vi "Pre-Build Custom Action.vi"(10 "Variant":variant) -> (0 "error out":errorcluster)   [LabVIEW 2017]
panel:
  out "States Out":string
  out "Current State":string
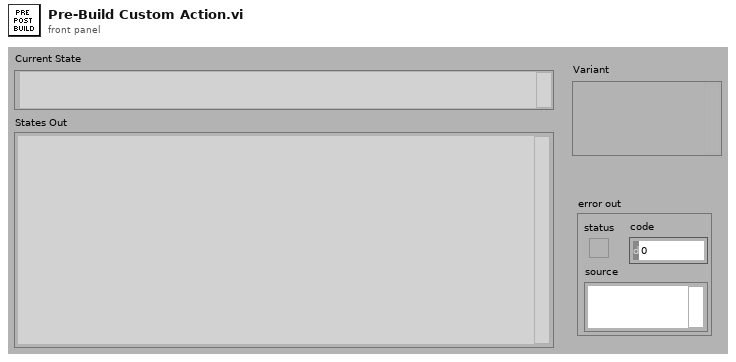
[diagram p1: front panel]
types:
  T1 = enum32{"Invalid", "Standard", "Closed", "Hidden", "Minimized", "Maximized"}
  T2 = enum32{"invalid app kind", "Development System", "Run Time System", "Student Edition", "Embedded LabVIEW", "Evaluation", "Custom"}
  T3 = cluster{"Core":cluster{"Current VI Reference":refnum<vi>, "Close Panel on Exit?":bool}, "Your Boolean data":bool, "Your string data":string}
  T4 = cluster{"Current VI Reference":refnum<vi>, "Close Panel on Exit?":bool}
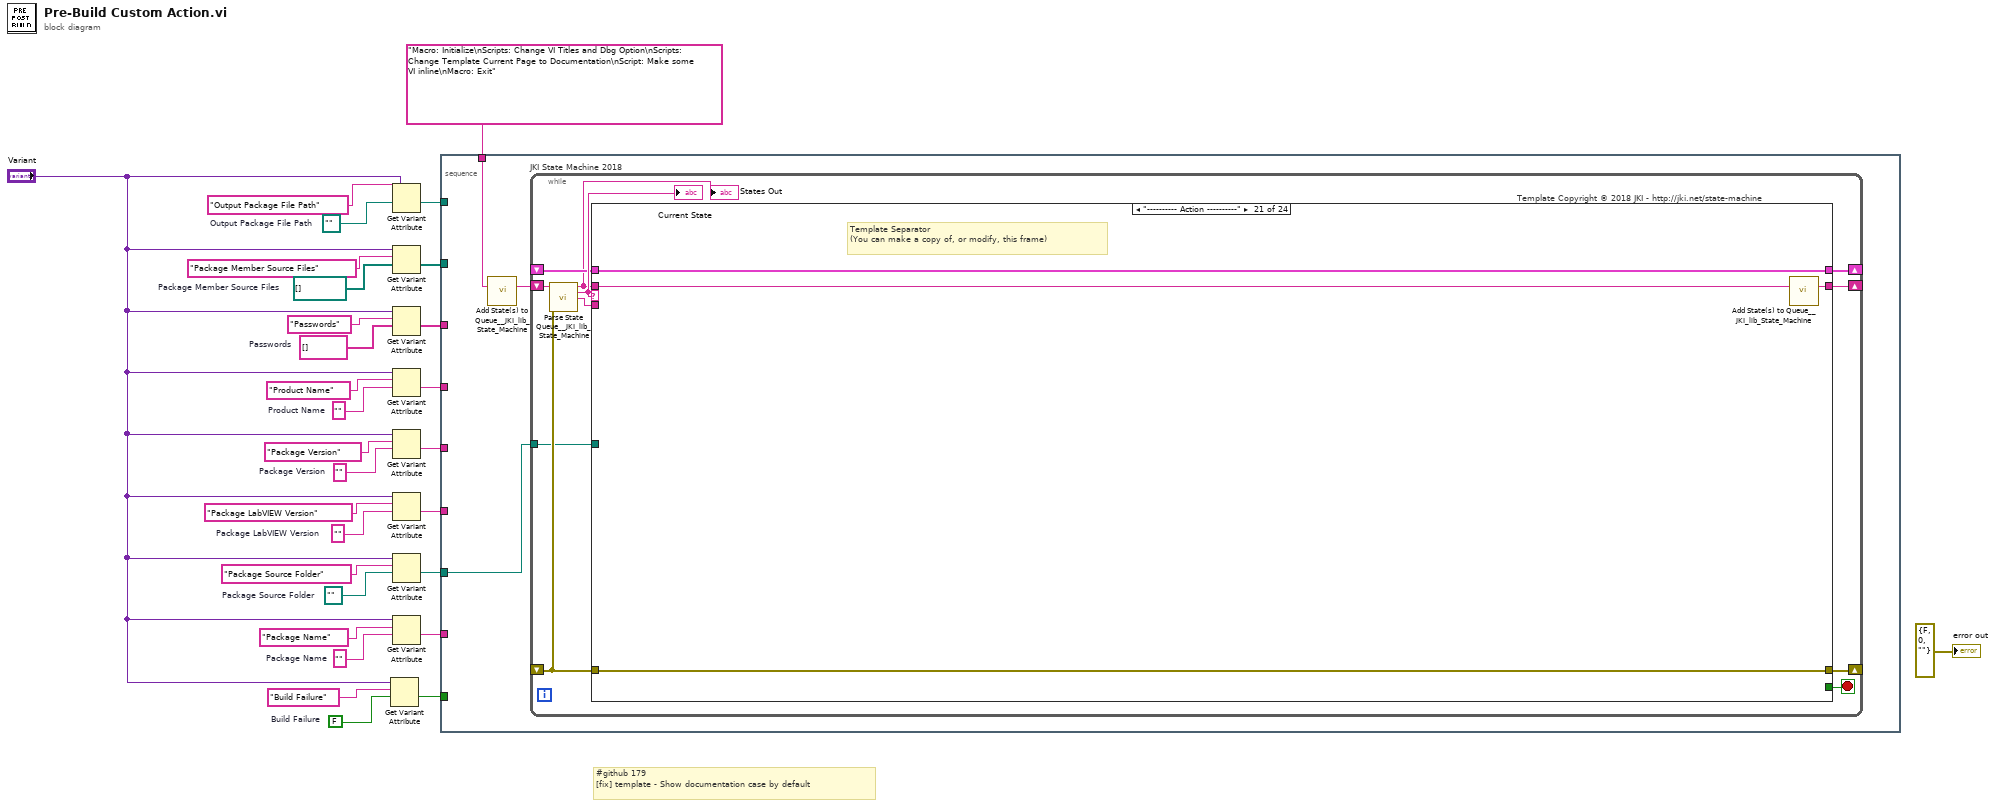
[diagram p0: block diagram]
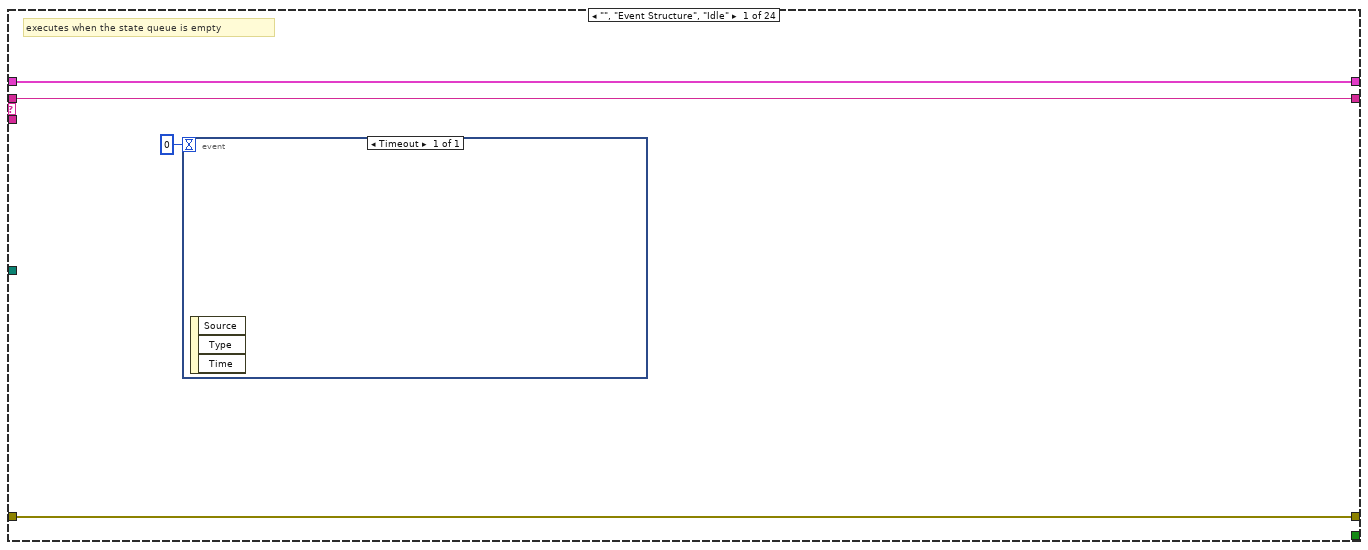
[diagram p2: hidden frame]
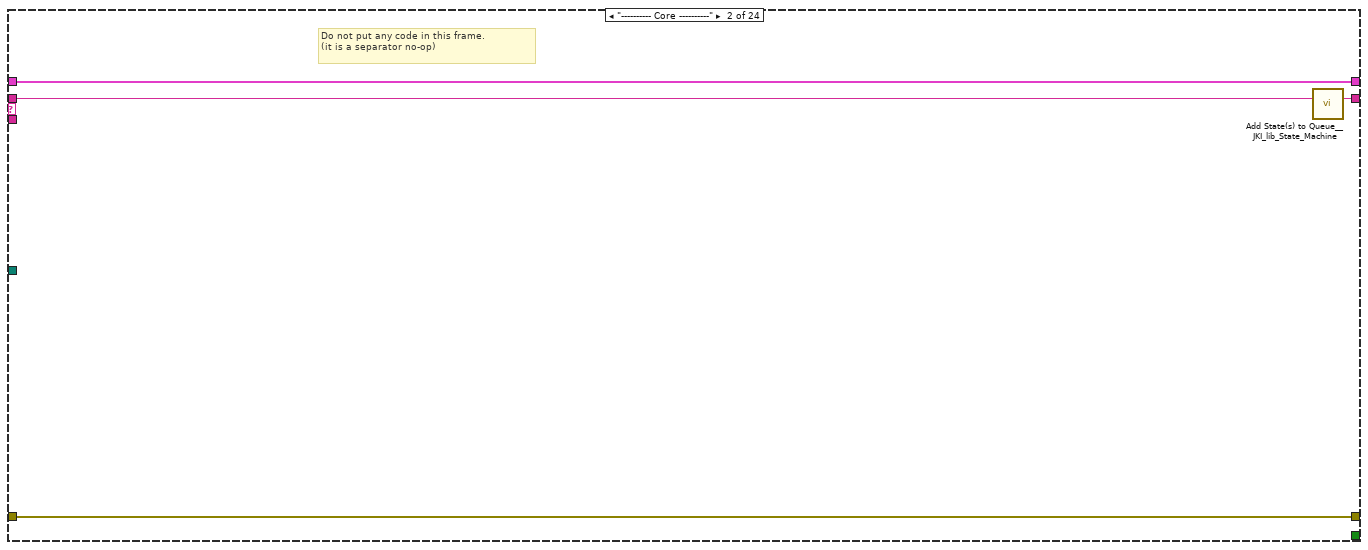
[diagram p3: hidden frame]
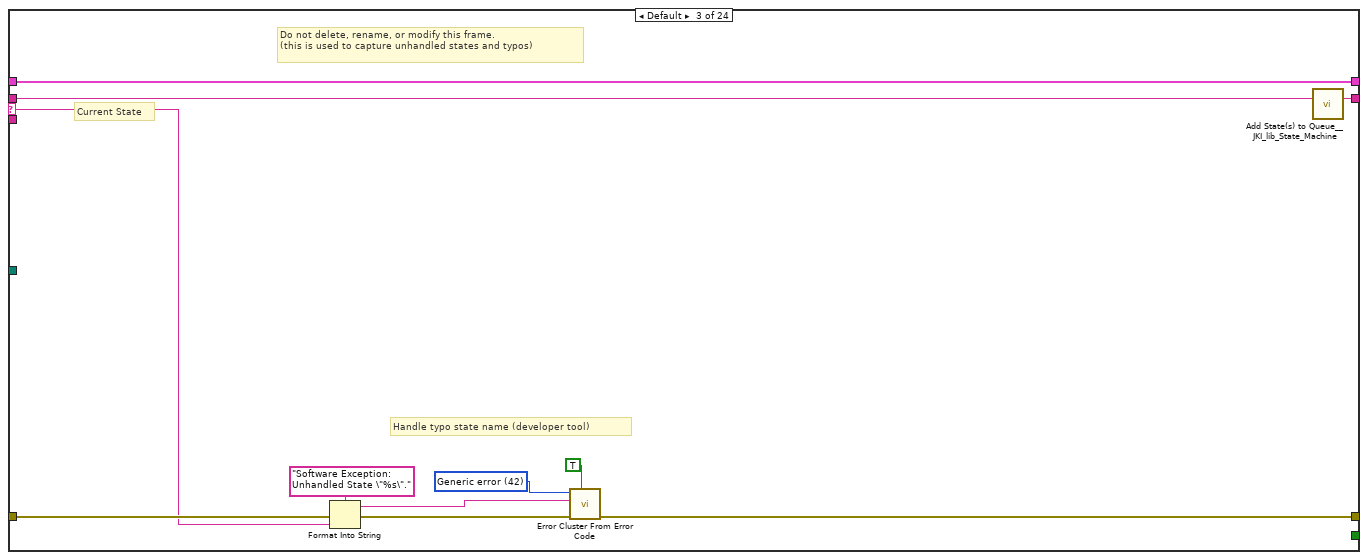
[diagram p4: hidden frame]
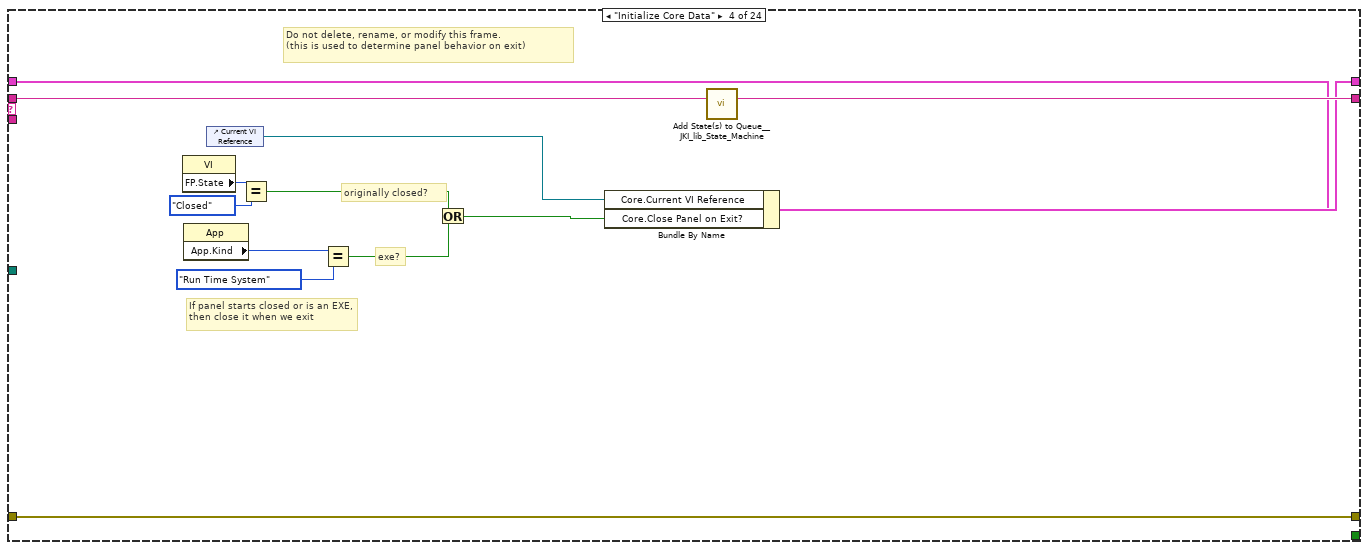
[diagram p5: hidden frame]
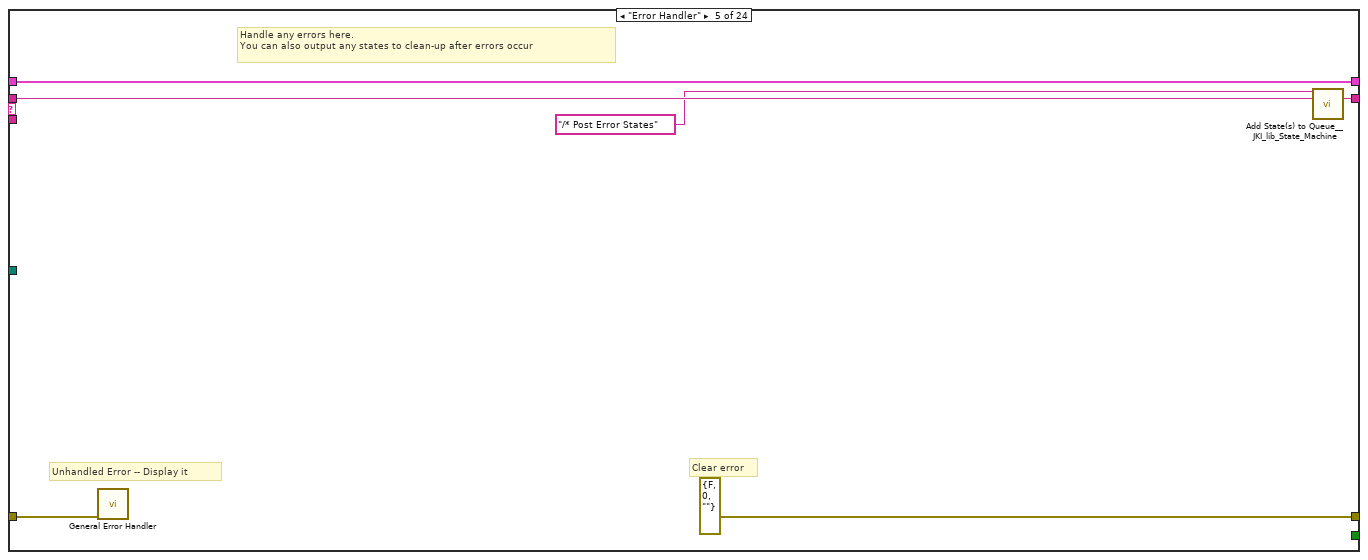
[diagram p6: hidden frame]
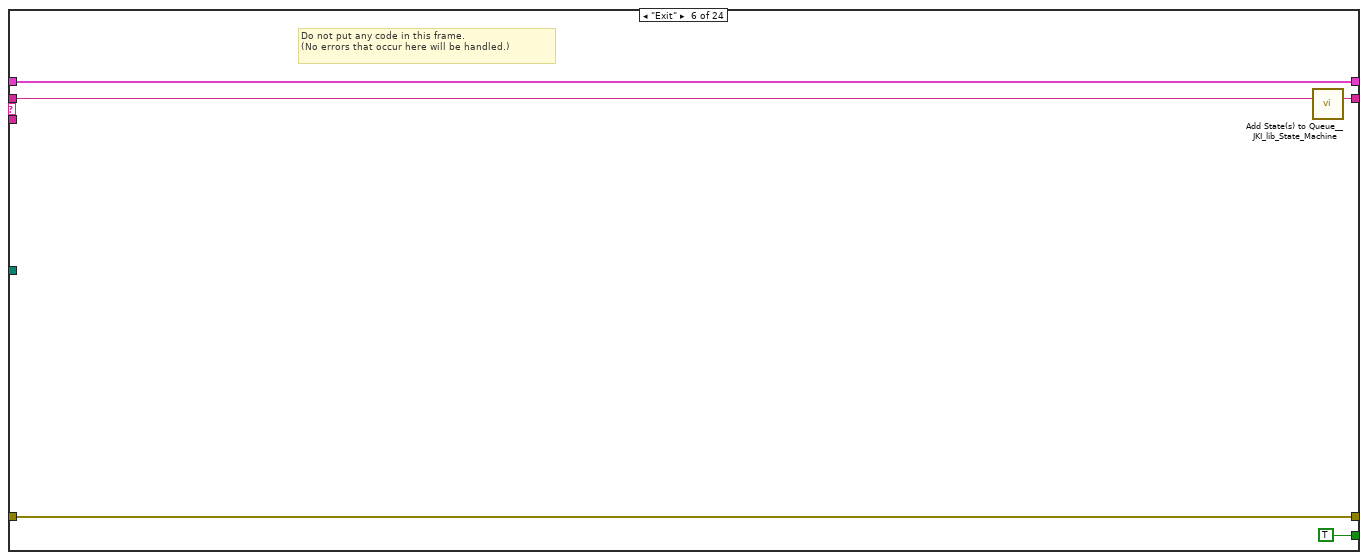
[diagram p7: hidden frame]
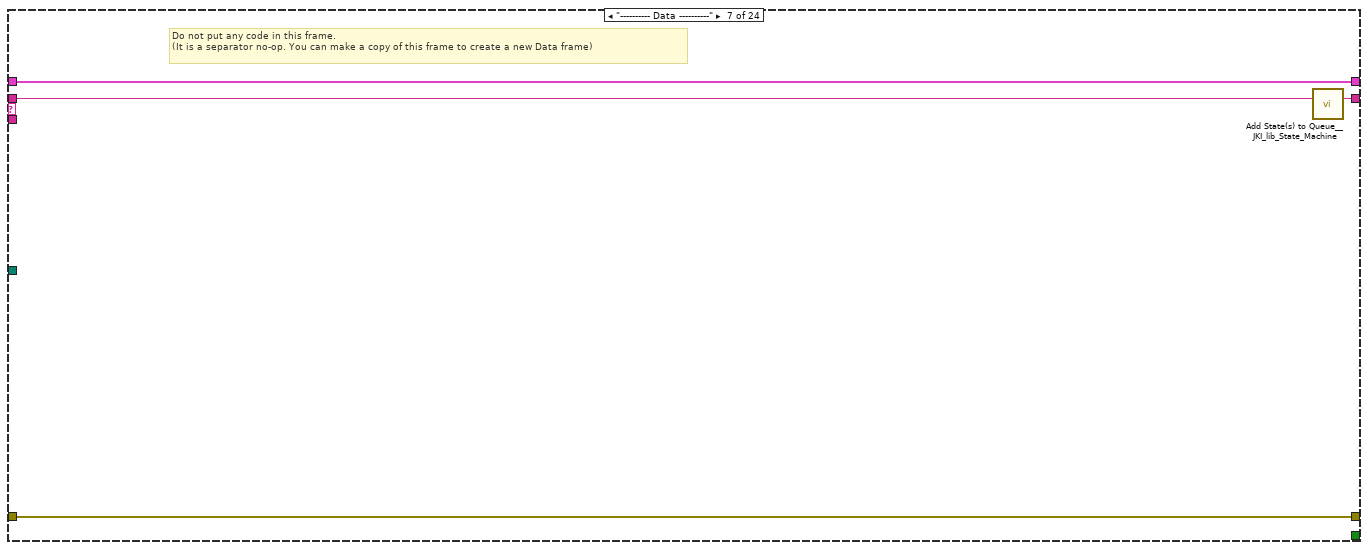
[diagram p8: hidden frame]
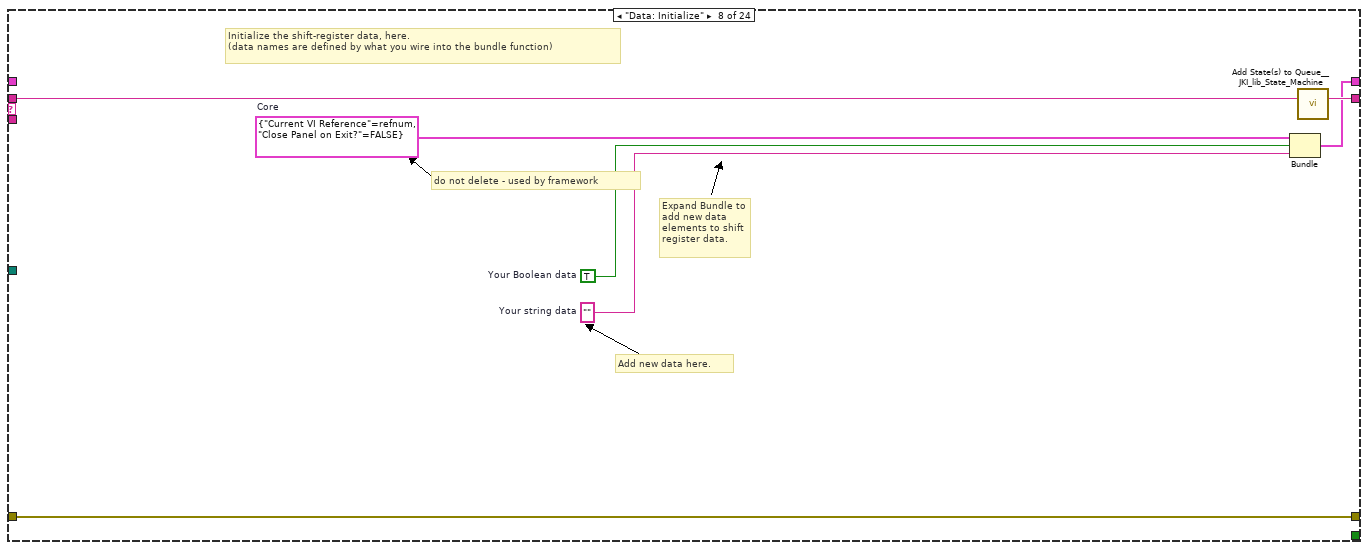
[diagram p9: hidden frame]
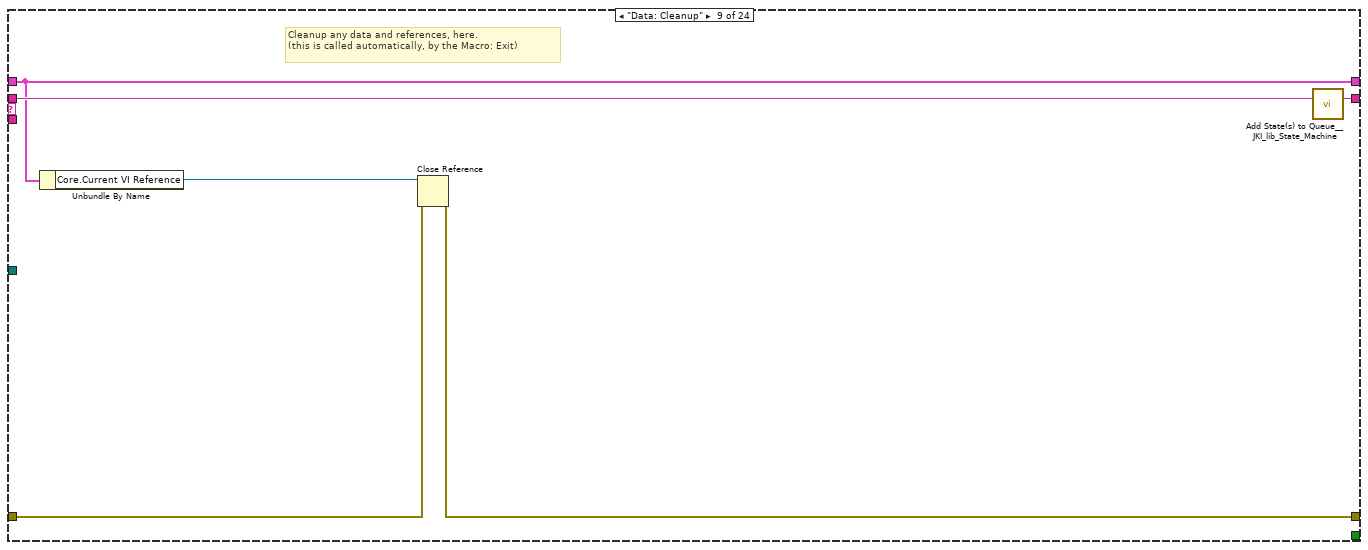
[diagram p10: hidden frame]
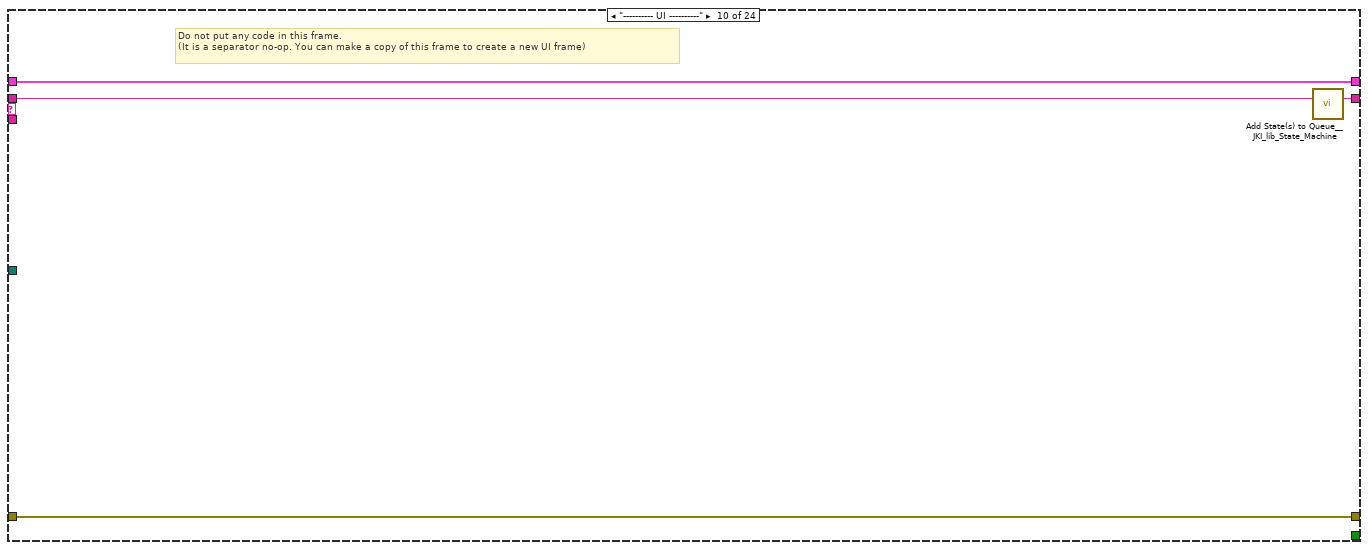
[diagram p11: hidden frame]
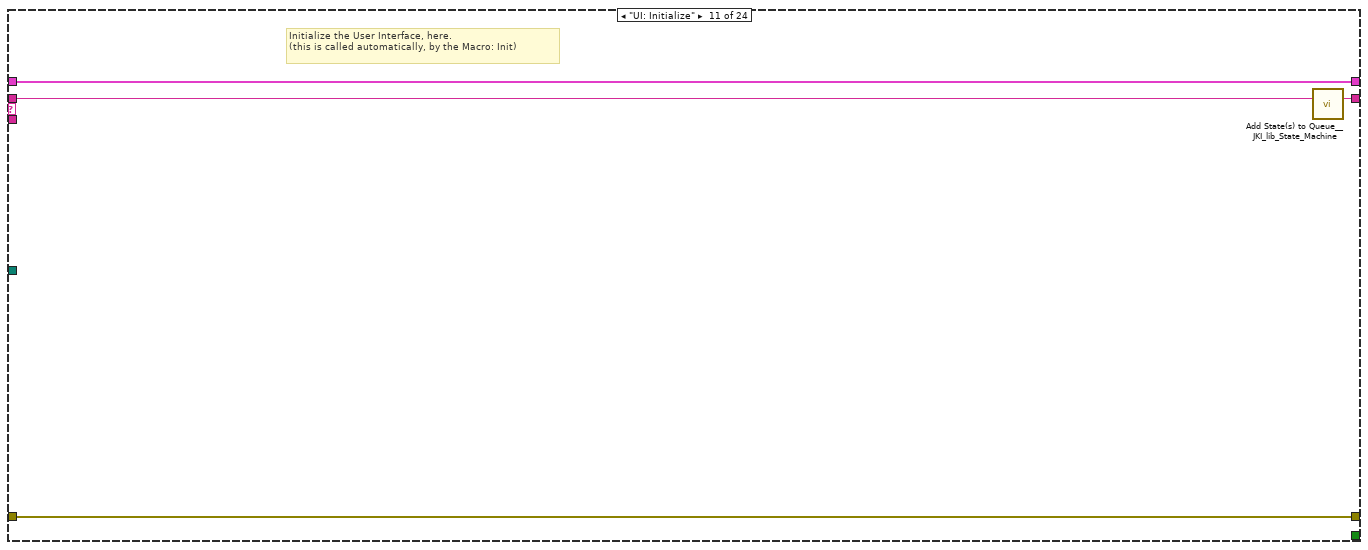
[diagram p12: hidden frame]
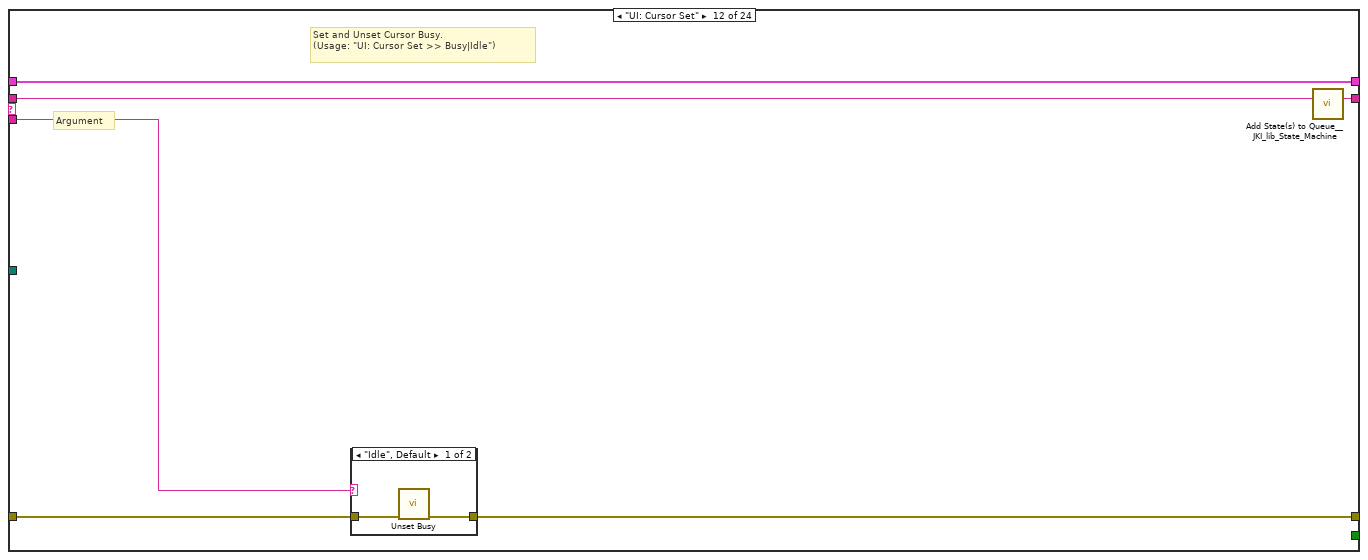
[diagram p13: hidden frame]
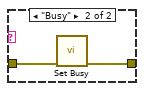
[diagram p14: hidden frame]
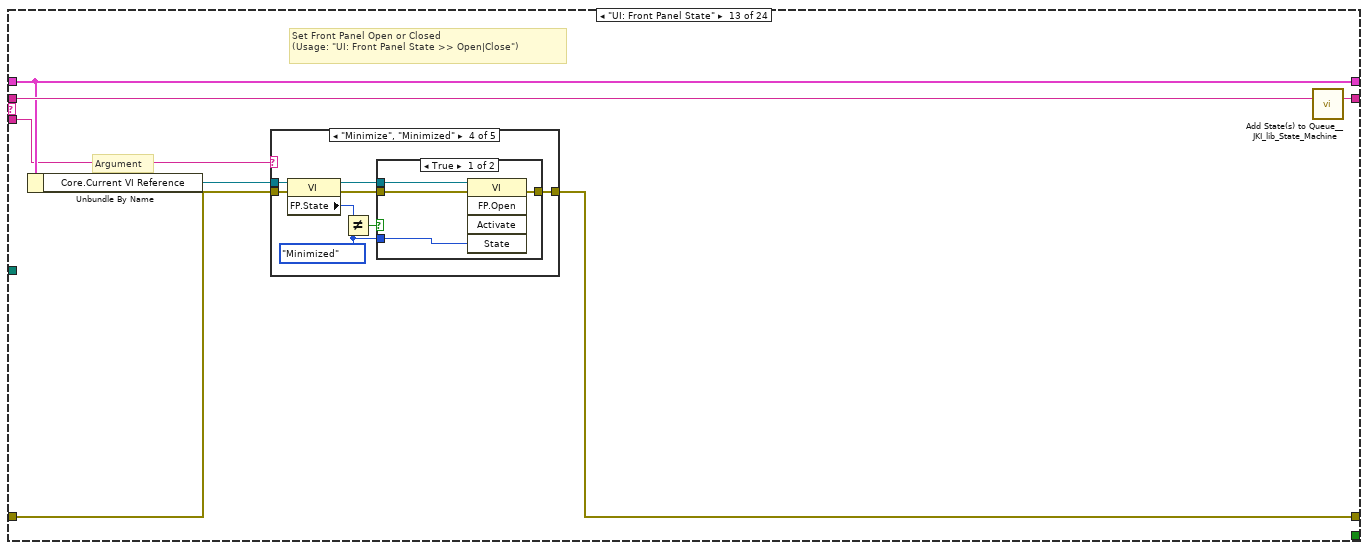
[diagram p15: hidden frame]
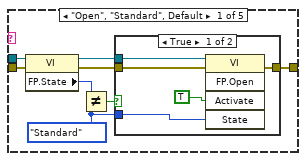
[diagram p16: hidden frame]
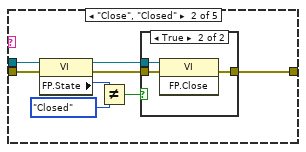
[diagram p18: hidden frame]
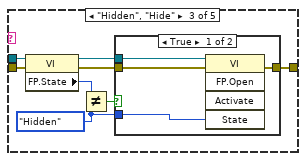
[diagram p20: hidden frame]
diagram:
  w4 = FALSE  # Build Failure
  w14 = path ""  # Package Source Folder
  w15 = ""  # Package Name
  w18 = ""  # Package LabVIEW Version
  w20 = ""  # Package Version
  w22 = ""  # Product Name
  w25 = string[] []  # Passwords
  w27 = path[] []  # Package Member Source Files
  w29 = path ""  # Output Package File Path
  # "#github 179\n[fix] template - Show documentation case by default"
  n1 = Get Variant Attribute(Variant="Variant", name="Build Failure", default value (empty Variant)=w4) -> (value=w2:bool)  [unwired: 1 in, 3 out]
  n2 = Get Variant Attribute(Variant="Variant", name="Output Package File Path", default value (empty Variant)=w29) -> (value=w13:path)  [unwired: 1 in, 3 out]
  n3 = Get Variant Attribute(Variant="Variant", name="Package Member Source Files", default value (empty Variant)=w27) -> (value=w12:path[])  [unwired: 1 in, 3 out]
  n4 = Get Variant Attribute(Variant="Variant", name="Passwords", default value (empty Variant)=w25) -> (value=w11:string[])  [unwired: 1 in, 3 out]
  n5 = Get Variant Attribute(Variant="Variant", name="Product Name", default value (empty Variant)=w22) -> (value=w10:string)  [unwired: 1 in, 3 out]
  n6 = Get Variant Attribute(Variant="Variant", name="Package Version", default value (empty Variant)=w20) -> (value=w9:string)  [unwired: 1 in, 3 out]
  n7 = Get Variant Attribute(Variant="Variant", name="Package LabVIEW Version", default value (empty Variant)=w18) -> (value=w8:string)  [unwired: 1 in, 3 out]
  n8 = Get Variant Attribute(Variant="Variant", name="Package Source Folder", default value (empty Variant)=w14) -> (value=w7:path)  [unwired: 1 in, 3 out]
  n9 = Get Variant Attribute(Variant="Variant", name="Package Name", default value (empty Variant)=w15) -> (value=w6:string)  [unwired: 1 in, 3 out]
  n10 = stacked-sequence {
    tunnel: w13 -> [_]
    tunnel: w12 -> [_]
    tunnel: w11 -> [_]
    tunnel: w10 -> [_]
    tunnel: w9 -> [_]
    tunnel: w8 -> [_]
    tunnel: w7 -> [w32]
    tunnel: w6 -> [_]
    tunnel: w2 -> [_]
    tunnel: "Macro: Initialize\nScripts: Change VI Titles and Dbg Option\nScripts: Change Template Current Page to Documentation\nScript: Make some VI inline\nMacro: Exit" -> [w31]
    frame #0 {
      n11 = call <vilib>:"Add State(s) to Queue__JKI_lib_State_Machine.vi"("State(s) in (\"\")"=w31) -> ("States Out"=w33:string)  [unwired: 14 in]
      n12 = while "JKI State Machine 2018" {
        shift-right: [w38] -> _
        shift-left: _ -> [w37]
        shift-right: [w41] -> _
        shift-left: _ -> [w36]
        shift-right: [w40] -> _
        shift-left: w33 -> [w42]
        tunnel: w32 -> [w35]
        stop <- w39 stop-if-true
        # "Template Copyright © 2018 JKI - http://jki.net/state-machine"
        n13 = call <vilib>:"Parse State Queue__JKI_lib_State_Machine.vi"("State Queue"=w42, "Error In (no error)"=w36) -> ("Remaining States"=w34:string, "Current State"=w44:string, "Arguments"=w43:string)  [unwired: 11 in]
        "Current State" <- w44
        "States Out" <- w34
        n14 = case shown="\"---------- Action ----------\"" w44 {
          selector: w44 -> [_ _ w53 _ _ _ _ _ _ _ _ _ _ _ _ _ _ _ _ _ _ _ _ _]
          tunnel: w34 -> [w47 w52 w57 w76 w82 w87 w91 w98 w104 w108 w112 w118 w129 w198 w203 w213 w217 w225 w265 w288 w312 w350 w375 w411]
          tunnel: w43 -> [_ _ _ _ _ _ _ _ _ _ _ w113 w123 _ _ _ _ _ _ _ _ w313 w357 w405]
          tunnel: w37 -> [w48 w49 w55 w69 w79 w85 w88 _ w99 w105 w110 w116 w125 w195 w200 w210 w214 w230 w268 w292 w309 w347 w372 w408]
          tunnel: [w46 w50 w59 w73 errorcluster {"status"=FALSE, "code"=0, "source"=""} ("error out") w84 w89 w95 w100 w106 w109 w114 w126 w196 w201 w211 w215 w231 w269 w293 w310 w348 w373 w409] -> w41
          tunnel: w36 -> [w46 w50 w58 w73 w78 w84 w89 w95 w101 w106 w109 w115 w127 w196 w201 w211 w215 w231 w269 w293 w310 w348 w373 w409]
          tunnel: [w47 w51 w56 w75 w81 w86 w90 w97 w103 w107 w111 w117 w128 w197 w202 w212 w216 w224 w264 w287 w311 w349 w374 w410] -> w40
          tunnel: [_ _ _ _ _ TRUE _ _ _ _ _ _ _ _ _ _ _ _ _ _ _ _ _ _] -> w39
          tunnel: [w48 w49 w55 w74 w79 w85 w88 w96 w99 w105 w110 w116 w125 w195 w200 w210 w214 w230 w268 w292 w309 w347 w372 w408] -> w38
          tunnel: w35 -> [_ _ _ _ _ _ _ _ _ _ _ _ _ _ _ _ _ w227 w267 w290 _ _ _ _]
          frame "", "Event Structure", "Idle" {
            # "executes when the state queue is empty"
            n15 = event shown="[0] Timeout" {
              selector: _ -> [_]
              dyn-events: _ -> [_]
              timeout: 0 -> [_]
              event Timeout {
                n16 = event-data() -> ()  [unwired: 1 in, 3 out]
              }
            }
          }
          frame "---------- Core ----------" {
            # "Do not put any code in this frame.\n(it is a separator no-op)"
            n17 = call <vilib>:"Add State(s) to Queue__JKI_lib_State_Machine.vi"("State(s) in (\"\")"=w52) -> ("States Out"=w51:string)  [unwired: 14 in]
          }
          frame Default {
            w62 = 42 items=["No error", "Argument error", "Memory is full", "Out of zone", "End of file", "File already open", "Generic file I/O error", "File not found", "File permission error", "Disk is full", "Duplicate path", "Too many files open", "System feature not enabled", "Resource file not found", "Cannot add resource", "Resource not found", "Image not found", "Image memory error", "Pen does not exist", "Config type invalid", "Config token not found", "Config parse error", "Config memory error", "Bad external code format", "Bad external code offset", "External code not present", "Null window", "Destroy window error", "Null menu", "Print aborted", "Bad print record", "Print driver error", "Windows error during printing", "Memory error during printing", "Print dialog error", "Generic print error", "Invalid device refnum", "Device not found", "Device parameter error", "Device unit error", "Cannot open device", "Device call aborted", "Generic error", "Cancelled by user", "Object ID too low", "Object ID too high", "Object not in heap", "Unknown heap", "Unknown object (invalid DefProc)", "Unknown object (DefProc not in table)", "Message out of range", "Invalid (null) method", "Unknown message", "Manager call not supported", "Bad address", "Network operation in progress", "Network operation timed out", "Connection is busy", "Network attribute not supported", "Network error", "Address in use", "System out of memory", "Connection aborted", "Connection refused", "Not connected", "Already connected", "Connection closed", "Initialization error (interapplication manager)", "Bad occurrence", "Wait on unbound occurrence handler", "Occurrence queue overflow", "Datalog type conflict", "Unused", "Unrecognized type (interapplication manager)", "Memory corrupt", "Failed to make temporary DLL", "Old CIN version", "Drag socket not found", "Failed to load drop-object", "Failed to register OLE object", "Failed to release OLE object", "Format specifier type mismatch", "Unknown format specifier", "Too few format specifiers", "Too many format specifiers", "Scan failed", "Newer CIN version", "Error converting to variant", "Runtime menu error", "Password tampered", "Variant attribute not found", "Incompatible variant data type", "Event data is not available", "Event Store is not present", "Occurrence is not found", "Event Queue is not created", "Event info is not available", "Refnum passed is NULL", "Error retrieving Class GUID", "Error retrieving CoClass GUID", "Error retrieving TypeLib GUID.", "Bad built application magic bytes.", "Specific driver is different from the specific driver associated with the Logical Name.", "There is no session opened to the class driver.", "Max Error", "MAX - Error with config objects", "MAX - Error loading configuration", "MAX - Group not supported"]
            # "Current State"
            # "Do not delete, rename, or modify this frame.\n(this is used to capture unhandled states and typos)"
            # "Handle typo state name (developer tool)"
            n18 = Format Into String(format string="Software Exception: Unhandled State \"%s\"." ("message"), error in=w58, w53) -> (resulting string=w61:string, error out=w60:errorcluster)  [unwired: 1 in]
            n19 = call <vilib>:"Error Cluster From Error Code.vi"("show call chain? (False)"=TRUE, "error in (no error)"=w60, "error message (\"\")"=w61, "error code (0)"=w62) -> ("error out"=w59:errorcluster)  [unwired: 5 in]
            n20 = call <vilib>:"Add State(s) to Queue__JKI_lib_State_Machine.vi"("State(s) in (\"\")"=w57) -> ("States Out"=w56:string)  [unwired: 14 in]
          }
          frame "Initialize Core Data" {
            # "Do not delete, rename, or modify this frame.\n(this is used to determine panel behavior on exit)"
            # "originally closed?"
            # "exe?"
            # "If panel starts closed or is an EXE, then close it when we exit"
            n21 = property class="VI"() -> ("FP.State"=w66:T1)  [unwired: 2 in, 2 out]
            n22 = property class="App"() -> ("App.Kind"=w72:T2)  [unwired: 2 in, 2 out]
            n23 = control-ref of="Current VI Reference"() -> (w67:refnum<vi>)
            n24 = Equal?(x=w66, y=T1."Closed" ("Front Panel Window:State")) -> (x = y?=w64:bool)
            n25 = Equal?(x=w72, y=T2."Run Time System" ("Application:Kind")) -> (x = y?=w70:bool)
            n26 = Or(x=w64, y=w70) -> (x .or. y?=w68:bool)
            n27 = Bundle By Name(cluster=w69, "Core.Current VI Reference"=w67, "Core.Close Panel on Exit?"=w68) -> (w74:T3)
            n28 = call <vilib>:"Add State(s) to Queue__JKI_lib_State_Machine.vi"("State(s) in (\"\")"=w76) -> ("States Out"=w75:string)  [unwired: 14 in]
          }
          frame "Error Handler" {
            # "Unhandled Error -- Display it"
            # "Handle any errors here.\nYou can also output any states to clean-up after errors occur"
            # "Clear error"
            n29 = call <vilib>:"General Error Handler.vi"("error in (no error)"=w78) -> ()  [unwired: 10 in, 5 out]
            n30 = call <vilib>:"Add State(s) to Queue__JKI_lib_State_Machine.vi"("State(s) in Front (\"\")"="/* Post Error States", "State(s) in (\"\")"=w82) -> ("States Out"=w81:string)  [unwired: 13 in]
          }
          frame "Exit" {
            # "Do not put any code in this frame.\n(No errors that occur here will be handled.)"
            n31 = call <vilib>:"Add State(s) to Queue__JKI_lib_State_Machine.vi"("State(s) in (\"\")"=w87) -> ("States Out"=w86:string)  [unwired: 14 in]
          }
          frame "---------- Data ----------" {
            # "Do not put any code in this frame.\n(It is a separator no-op. You can make a copy of this frame to create a new Data frame)"
            n32 = call <vilib>:"Add State(s) to Queue__JKI_lib_State_Machine.vi"("State(s) in (\"\")"=w91) -> ("States Out"=w90:string)  [unwired: 14 in]
          }
          frame "Data: Initialize" {
            w92 = T4 {"Current VI Reference"=refnum, "Close Panel on Exit?"=FALSE}  # Core
            w94 = TRUE  # Your Boolean data
            w93 = ""  # Your string data
            # "do not delete - used by framework"
            # "Expand Bundle to add new data elements to shift register data."
            # "Add new data here."
            # "Initialize the shift-register data, here.\n(data names are defined by what you wire into the bundle function)"
            n33 = Bundle("Core"=w92, "Your Boolean data"=w94, "Your string data"=w93) -> (w96:T3)  [unwired: 1 in]
            n34 = call <vilib>:"Add State(s) to Queue__JKI_lib_State_Machine.vi"("State(s) in (\"\")"=w98) -> ("States Out"=w97:string)  [unwired: 14 in]
          }
          frame "Data: Cleanup" {
            # "Cleanup any data and references, here.\n(this is called automatically, by the Macro: Exit)"
            n35 = Unbundle By Name(w99) -> ("Core.Current VI Reference"=w102:refnum<vi>)
            n36 = Close Reference(reference=w102, error in (no error)=w101) -> (error out=w100:errorcluster)
            n37 = call <vilib>:"Add State(s) to Queue__JKI_lib_State_Machine.vi"("State(s) in (\"\")"=w104) -> ("States Out"=w103:string)  [unwired: 14 in]
          }
          frame "---------- UI ----------" {
            # "Do not put any code in this frame.\n(It is a separator no-op. You can make a copy of this frame to create a new UI frame)"
            n38 = call <vilib>:"Add State(s) to Queue__JKI_lib_State_Machine.vi"("State(s) in (\"\")"=w108) -> ("States Out"=w107:string)  [unwired: 14 in]
          }
          frame "UI: Initialize" {
            # "Initialize the User Interface, here.\n(this is called automatically, by the Macro: Init)"
            n39 = call <vilib>:"Add State(s) to Queue__JKI_lib_State_Machine.vi"("State(s) in (\"\")"=w112) -> ("States Out"=w111:string)  [unwired: 14 in]
          }
          frame "UI: Cursor Set" {
            # "Argument"
            # "Set and Unset Cursor Busy.\n(Usage: \"UI: Cursor Set >> Busy|Idle\")"
            n40 = case shown="\"Idle\", Default" w113 {
              tunnel: w115 -> [w120 w122]
              tunnel: [w119 w121] -> w114
              frame "Idle", Default {
                n41 = call <vilib>:"Unset Busy.vi"("error in (no error)"=w120) -> ("error out"=w119:errorcluster)  [unwired: 10 in]
              }
              frame "Busy" {
                n42 = call <vilib>:"Set Busy.vi"("error in (no error)"=w122) -> ("error out"=w121:errorcluster)  [unwired: 9 in, 1 out]
              }
            }
            n43 = call <vilib>:"Add State(s) to Queue__JKI_lib_State_Machine.vi"("State(s) in (\"\")"=w118) -> ("States Out"=w117:string)  [unwired: 14 in]
          }
          frame "UI: Front Panel State" {
            # "Argument"
            # "Set Front Panel Open or Closed\n(Usage: \"UI: Front Panel State >> Open|Close\")"
            n44 = Unbundle By Name(w125) -> ("Core.Current VI Reference"=w124:refnum<vi>)
            n45 = case shown="\"Minimize\", \"Minimized\"" w123 {
              tunnel: w127 -> [w135 w150 w161 w174 w187]
              tunnel: [w137 w151 w163 w176 w189] -> w126
              tunnel: w124 -> [w136 w148 w162 w175 w188]
              frame "Open", "Standard", Default {
                w130 = T1."Standard" ("State")
                n46 = property class="VI"(reference=w136, error in=w135) -> (reference out=w133:refnum<vi>, error out=w134:errorcluster, "FP.State"=w132:T1)
                n47 = Not Equal?(x=w132, y=w130) -> (x != y?=w131:bool)
                n48 = case shown="True" w131 {
                  tunnel: [w141 w143] -> w137
                  tunnel: w134 -> [w140 w143]
                  tunnel: w133 -> [w139 _]
                  tunnel: w130 -> [w138 _]
                  frame True {
                    n49 = invoke class="VI" method="FP.Open"(reference=w139, error in=w140, "Activate"=TRUE, "State"=w138) -> (error out=w141:errorcluster)  [unwired: 1 in, 4 out]
                  }
                  frame False {
                  }
                }
              }
              frame "Close", "Closed" {
                n50 = property class="VI"(reference=w148, error in=w150) -> (reference out=w147:refnum<vi>, error out=w149:errorcluster, "FP.State"=w145:T1)
                n51 = Not Equal?(x=w145, y=T1."Closed" ("Front Panel Window:State")) -> (x != y?=w144:bool)
                n52 = case shown="True" w144 {
                  tunnel: [w152 w155] -> w151
                  tunnel: w149 -> [w152 w154]
                  tunnel: w147 -> [_ w153]
                  frame False {
                  }
                  frame True {
                    n53 = invoke class="VI" method="FP.Close"(reference=w153, error in=w154) -> (error out=w155:errorcluster)  [unwired: 1 in, 2 out]
                  }
                }
              }
              frame "Hidden", "Hide" {
                w156 = T1."Hidden" ("State")
                n54 = property class="VI"(reference=w162, error in=w161) -> (reference out=w159:refnum<vi>, error out=w160:errorcluster, "FP.State"=w158:T1)
                n55 = Not Equal?(x=w158, y=w156) -> (x != y?=w157:bool)
                n56 = case shown="True" w157 {
                  tunnel: [w167 w168] -> w163
                  tunnel: w160 -> [w166 w168]
                  tunnel: w159 -> [w165 _]
                  tunnel: w156 -> [w164 _]
                  frame True {
                    n57 = invoke class="VI" method="FP.Open"(reference=w165, error in=w166, "State"=w164) -> (error out=w167:errorcluster)  [unwired: 2 in, 4 out]
                  }
                  frame False {
                  }
                }
              }
              frame "Minimize", "Minimized" {
                w169 = T1."Minimized" ("State")
                n58 = property class="VI"(reference=w175, error in=w174) -> (reference out=w172:refnum<vi>, error out=w173:errorcluster, "FP.State"=w171:T1)
                n59 = Not Equal?(x=w171, y=w169) -> (x != y?=w170:bool)
                n60 = case shown="True" w170 {
                  tunnel: [w180 w181] -> w176
                  tunnel: w173 -> [w179 w181]
                  tunnel: w172 -> [w178 _]
                  tunnel: w169 -> [w177 _]
                  frame True {
                    n61 = invoke class="VI" method="FP.Open"(reference=w178, error in=w179, "State"=w177) -> (error out=w180:errorcluster)  [unwired: 2 in, 4 out]
                  }
                  frame False {
                  }
                }
              }
              frame "Maximize", "Maximized" {
                w182 = T1."Maximized" ("State")
                n62 = property class="VI"(reference=w188, error in=w187) -> (reference out=w185:refnum<vi>, error out=w186:errorcluster, "FP.State"=w184:T1)
                n63 = Not Equal?(x=w184, y=w182) -> (x != y?=w183:bool)
                n64 = case shown="True" w183 {
                  tunnel: [w193 w194] -> w189
                  tunnel: w186 -> [w192 w194]
                  tunnel: w185 -> [w191 _]
                  tunnel: w182 -> [w190 _]
                  frame True {
                    n65 = invoke class="VI" method="FP.Open"(reference=w191, error in=w192, "State"=w190) -> (error out=w193:errorcluster)  [unwired: 2 in, 4 out]
                  }
                  frame False {
                  }
                }
              }
            }
            n66 = call <vilib>:"Add State(s) to Queue__JKI_lib_State_Machine.vi"("State(s) in (\"\")"=w129) -> ("States Out"=w128:string)  [unwired: 14 in]
          }
          frame "---------- Macro ----------" {
            # "Do not put any code in this frame.\n(It is a separator no-op. You can make a copy of this frame to create a new Macro frame)"
            n67 = call <vilib>:"Add State(s) to Queue__JKI_lib_State_Machine.vi"("State(s) in (\"\")"=w198) -> ("States Out"=w197:string)  [unwired: 14 in]
          }
          frame "Macro: Initialize" {
            w199 = "Data: Initialize\nInitialize Core Data\nUI: Initialize\nUI: Front Panel State >> Open"  # Data: Initialize Initialize Core Data UI: Initialize UI: Front Panel State >> Open
            # "Initialization Macro\n(This is called once, when the VI starts)"
            n68 = call <vilib>:"Add State(s) to Queue__JKI_lib_State_Machine.vi"("State(s) in Front (\"\")"=w199, "State(s) in (\"\")"=w203) -> ("States Out"=w202:string)  [unwired: 13 in]
          }
          frame "Macro: Exit" {
            # "Exit Macro\n(This is called once, when the VI exits)"
            n69 = Unbundle By Name(w210) -> ("Core.Close Panel on Exit?"=w209:bool)
            n70 = Select(t="UI: Front Panel State >> Close", s=w209, f="") -> (s? t:f=w206:string)
            n71 = call <vilib>:"Add State(s) to Queue__JKI_lib_State_Machine.vi"("State(s) in (\"\")"=w206, "State(s) at Back (\"\")"="Data: Cleanup\nExit") -> ("States Out"=w204:string)  [unwired: 13 in]
            n72 = call <vilib>:"Add State(s) to Queue__JKI_lib_State_Machine.vi"("State(s) in Front (\"\")"=w204, "State(s) in (\"\")"=w213) -> ("States Out"=w212:string)  [unwired: 13 in]
          }
          frame "---------- Scripts ----------" {
            # "Template Separator\n(You can make a copy of, or modify, this frame)"
            n73 = call <vilib>:"Add State(s) to Queue__JKI_lib_State_Machine.vi"("State(s) in (\"\")"=w217) -> ("States Out"=w216:string)  [unwired: 14 in]
          }
          frame "Scripts: Change VI Titles and Dbg Option" {
            n74 = Empty String/Path?(string/path=w227) -> (empty?=w226:bool)
            n75 = case shown="True" w226 {
              tunnel: [w242 w243] -> w229
              tunnel: w227 -> [w242 _]
              frame False {
              }
              frame True {
                n76 = Current VI's Path() -> (path=w245:path)
                n77 = Strip Path(path=w245) -> (stripped path=w244:path)  [unwired: 1 out]
                n78 = Strip Path(path=w244) -> (stripped path=w243:path)  [unwired: 1 out]
              }
            }
            n79 = for {
              tunnel: w229 -> [w235]
              tunnel: string[] ["_vipm_actions", "_test", "_support", "resource", "_xnode", "_tool"] ("Folders to Exclude") -> [w234]
              tunnel: string[] ["*.vi", "*.vim", "*.vit"] -> [w233] mode=indexing
              tunnel: [w232] -> w219 mode=concatenating
              n80 = call <vilib>:"Recursive File List.vi"("Folders to Exclude"=w234, "pattern"=w233, "Folder Path"=w235) -> ("All Files in Dir"=w232:path[])  [unwired: 4 in, 4 out]
            }
            n81 = Current VI's Path() -> (path=w223:path)
            n82 = Search 1D Array(1D array=w219, element=w223) -> (index of element=w222:i32)  [unwired: 1 in]
            n83 = Delete From Array(array=w219, index=w222) -> (array with subset deleted=w221:path[])  [unwired: 1 in, 1 out]
            n84 = for {
              tunnel: w221 -> [w238] mode=indexing
              shift-right: [w240] -> w224
              shift-left: w225 -> [w241]
              tunnel: "Action: Change Title and Disable Dbg Option" ("State") -> [w236]
              n85 = Path To String(path=w238) -> (string=w237:string)
              n86 = call <vilib>:"Build State String with Arguments__JKI_lib_State_Machine.vi"("Arguments (\"\")"=w237, "State"=w236) -> ("State with Arguments"=w239:string)  [unwired: 4 in]
              n87 = call <vilib>:"Add State(s) to Queue__JKI_lib_State_Machine.vi"("State(s) in Front (\"\")"=w239, "State(s) in (\"\")"=w241) -> ("States Out"=w240:string)  [unwired: 13 in]
            }
          }
          frame "Scripts: Change Template Current Page to Documentation" {
            n88 = Empty String/Path?(string/path=w267) -> (empty?=w266:bool)
            n89 = case shown="True" w266 {
              tunnel: [w279 w280] -> w248
              tunnel: w267 -> [w279 _]
              frame False {
              }
              frame True {
                n90 = Current VI's Path() -> (path=w284:path)
                n91 = Strip Path(path=w284) -> (stripped path=w283:path)  [unwired: 1 out]
                n92 = Strip Path(path=w283) -> (stripped path=w282:path)  [unwired: 1 out]
                n93 = Build Path(base path=w282, name or relative path="user.lib") -> (appended path=w280:path)
              }
            }
            n94 = Strip Path(path=w248) -> (stripped path=w249:path)  [unwired: 1 out]
            n95 = Build Path(base path=w249, name or relative path=path "templates/Communicable State Machine(CSM)") -> (appended path=w263:path)
            n96 = call <vilib>:"Recursive File List.vi"("pattern"="CSM - *Template*.vi" ("name or relative path"), "Folder Path"=w248) -> ("error out"=w257:errorcluster, "All Files in Dir"=w258:path[])  [unwired: 5 in, 3 out]
            n97 = List Folder(path=w263, pattern="*.vit", error in=w257) -> (path out=w252:path, filenames=w259:string[], error out=w254:errorcluster)  [unwired: 1 in, 1 out]
            n98 = List Folder(path=w252, pattern="*.vi", error in=w254) -> (filenames=w260:string[], error out=w255:errorcluster)  [unwired: 1 in, 2 out]
            n99 = Build Array (concatenate)(w259, w260) -> (w261:string[])
            n100 = for {
              tunnel: w261 -> [w272] mode=indexing
              tunnel: [w271] -> w262 mode=indexing
              tunnel: w263 -> [w270]
              n101 = Build Path(base path=w270, name or relative path=w272) -> (appended path=w271:path)
            }
            n102 = call <vilib>:"Clear Errors.vi"("error in (no error)"=w255) -> ()  [unwired: 5 in, 2 out]
            n103 = Build Array (concatenate)(w258, w262) -> (w247:path[])
            n104 = for {
              tunnel: w247 -> [w275] mode=indexing
              shift-right: [w277] -> w264
              shift-left: w265 -> [w278]
              tunnel: "Action: Change CSM Documentation Case to Front" ("State") -> [w273]
              n105 = Path To String(path=w275) -> (string=w274:string)
              n106 = call <vilib>:"Build State String with Arguments__JKI_lib_State_Machine.vi"("Arguments (\"\")"=w274, "State"=w273) -> ("State with Arguments"=w276:string)  [unwired: 4 in]
              n107 = call <vilib>:"Add State(s) to Queue__JKI_lib_State_Machine.vi"("State(s) in Front (\"\")"=w276, "State(s) in (\"\")"=w278) -> ("States Out"=w277:string)  [unwired: 13 in]
            }
          }
          frame "Script: Make some VI inline" {
            n108 = Empty String/Path?(string/path=w290) -> (empty?=w289:bool)
            n109 = case shown="True" w289 {
              tunnel: [w303 w304] -> w291
              tunnel: w290 -> [w303 _]
              frame False {
              }
              frame True {
                n110 = Current VI's Path() -> (path=w308:path)
                n111 = Strip Path(path=w308) -> (stripped path=w307:path)  [unwired: 1 out]
                n112 = Strip Path(path=w307) -> (stripped path=w306:path)  [unwired: 1 out]
                n113 = Build Path(base path=w306, name or relative path="user.lib") -> (appended path=w304:path)
              }
            }
            n114 = for {
              tunnel: string[] ["Build State String with Arguments++.vi", "Add State(s) to Queue By BOOL", "CSM - Convert Data to HexStr.vi", "CSM - Convert HexStr to Data.vi", "CSM - Broadcast Status Change.vi", "CSM - Mark As Worker Module.vi", "CSM - Compact Multiple States.vi", "CSM - Register Status Change.vi", "CSM - Unregister Status Change.vi", "CSM - Check If Module Exists.vi", "CSM - List Modules.vi", "CSM - Get New State Notifier Event.vi"] -> [w296] mode=indexing
              tunnel: w291 -> [w295]
              tunnel: [w294] -> w286 mode=concatenating
              n115 = call <vilib>:"Recursive File List.vi"("pattern"=w296, "Folder Path"=w295) -> ("All Files in Dir"=w294:path[])  [unwired: 5 in, 4 out]
            }
            n116 = for {
              tunnel: w286 -> [w298] mode=indexing
              shift-right: [w301] -> w287
              shift-left: w288 -> [w302]
              n117 = Path To String(path=w298) -> (string=w297:string)
              n118 = call <vilib>:"Build State String with Arguments__JKI_lib_State_Machine.vi"("Arguments (\"\")"=w297, "State"="Action: Make VI inline") -> ("State with Arguments"=w299:string)  [unwired: 4 in]
              n119 = call <vilib>:"Add State(s) to Queue__JKI_lib_State_Machine.vi"("State(s) in Front (\"\")"=w299, "State(s) in (\"\")"=w302) -> ("States Out"=w301:string)  [unwired: 13 in]
            }
          }
          frame "---------- Action ----------" {
            # "Template Separator\n(You can make a copy of, or modify, this frame)"
            n120 = call <vilib>:"Add State(s) to Queue__JKI_lib_State_Machine.vi"("State(s) in (\"\")"=w312) -> ("States Out"=w311:string)  [unwired: 14 in]
          }
          frame "Action: Change Title and Disable Dbg Option" {
            w318 = FALSE ("Execution:Allow Debugging")
            w334 = "(CSM)" ("string")
            n121 = String To Path(string=w313) -> (path=w314:path)
            n122 = Strip Path(path=w314) -> (name=w330:string)  [unwired: 1 out]
            n123 = Open VI Reference(vi path=w314) -> (vi reference=w341:refnum<vi>, error out=w343:errorcluster)  [unwired: 5 in]
            n124 = Match Pattern(string=w330, regular expression=".vi[m]?$") -> (before substring=w336:string)  [unwired: 1 in, 3 out]
            n125 = property class="VI"(reference=w341, error in=w343) -> (reference out=w340:refnum<vi>, error out=w342:errorcluster, "Front Panel.Title"=w321:string)
            n126 = Match Pattern(string=w321, regular expression=w334) -> (offset past match=w338:i32)  [unwired: 1 in, 3 out]
            n127 = Greater Or Equal To 0?(x=w338) -> (x >= 0?=w337:bool)
            n128 = Select(t=w321, s=w337, f=w336) -> (s? t:f=w335:string)
            n129 = Search and Replace String(replace all?=TRUE ("replace all? (F)"), input string=w335, search string=w334) -> (result string=w332:string)  [unwired: 5 in, 3 out]
            n130 = call <vilib>:"Trim Whitespace.vi"("string"=w332) -> ("trimmed string"=w329:string)  [unwired: 1 in]
            n131 = Concatenate Strings(w329, " (CSM)" ("string")) -> (w320:string)
            n132 = property class="VI"(reference=w340, error in=w342, "Front Panel.Title"=w320) -> (reference out=w325:refnum<vi>, error out=w322:errorcluster)
            n133 = property class="VI"(reference=w325, error in=w322) -> (reference out=w324:refnum<vi>, error out=w323:errorcluster, "Exec.AllowDebug"=w319:bool)
            n134 = property class="VI"(reference=w324, error in=w323, "Exec.AllowDebug"=w318) -> (error out=w328:errorcluster)  [unwired: 1 out]
            n135 = Not Equal?(x=w321, y=w320) -> (x != y?=w317:bool)
            n136 = Not Equal?(x=w319, y=w318) -> (x != y?=w316:bool)
            n137 = Or(x=w317, y=w316) -> (x .or. y?=w315:bool)
            n138 = call <vilib>:"Clear Errors.vi"("error in (no error)"=w328) -> ("error out"=w326:errorcluster)  [unwired: 5 in, 1 out]
            n139 = Merge Errors(w322, w326) -> (w327:errorcluster)
            n140 = case shown="True" w315 {
              tunnel: [w351 w356] -> w346
              tunnel: [w352 w355] -> w345
              tunnel: w327 -> [w351 w354]
              tunnel: w325 -> [w352 w353]
              frame False {
              }
              frame True {
                n141 = invoke class="VI" method="Save.Instrument"(reference=w353, error in=w354) -> (reference out=w355:refnum<vi>, error out=w356:errorcluster)  [unwired: 4 in, 4 out]
              }
            }
            n142 = Close Reference(reference=w345, error in (no error)=w346) -> (error out=w331:errorcluster)
            n143 = Bundle("name"=w330, "error out"=w331) -> ()  [unwired: 1 in, 1 out]
            n144 = call <vilib>:"Clear Errors.vi"("error in (no error)"=w331) -> ()  [unwired: 5 in, 2 out]
            n145 = call <vilib>:"Add State(s) to Queue__JKI_lib_State_Machine.vi"("State(s) in (\"\")"=w350) -> ("States Out"=w349:string)  [unwired: 14 in]
          }
          frame "Action: Make VI inline" {
            w360 = TRUE ("Execution:Allow Debugging")
            n146 = String To Path(string=w357) -> (path=w358:path)
            n147 = Open VI Reference(vi path=w358) -> (vi reference=w368:refnum<vi>, error out=w369:errorcluster)  [unwired: 5 in]
            n148 = property class="VI"(reference=w368, error in=w369) -> (reference out=w363:refnum<vi>, error out=w362:errorcluster, "ExecInlining"=w361:bool)
            n149 = property class="VI"(reference=w363, error in=w362, "ExecInlining"=w360) -> (error out=w366:errorcluster)  [unwired: 1 out]
            n150 = call <vilib>:"Clear Errors.vi"("error in (no error)"=w366) -> ("error out"=w364:errorcluster)  [unwired: 5 in, 1 out]
            n151 = Not Equal?(x=w361, y=w360) -> (x != y?=w359:bool)
            n152 = Merge Errors(w369, w364) -> (w365:errorcluster)
            n153 = case shown="True" w359 {
              tunnel: [w376 w381] -> w371
              tunnel: [w377 w380] -> w370
              tunnel: w365 -> [w376 w379]
              tunnel: w368 -> [w377 w378]
              frame False {
              }
              frame True {
                n154 = invoke class="VI" method="Save.Instrument"(reference=w378, error in=w379) -> (reference out=w380:refnum<vi>, error out=w381:errorcluster)  [unwired: 4 in, 4 out]
              }
            }
            n155 = Close Reference(reference=w370, error in (no error)=w371) -> (error out=w367:errorcluster)
            n156 = call <vilib>:"Clear Errors.vi"("error in (no error)"=w367) -> ()  [unwired: 5 in, 2 out]
            n157 = call <vilib>:"Add State(s) to Queue__JKI_lib_State_Machine.vi"("State(s) in (\"\")"=w375) -> ("States Out"=w374:string)  [unwired: 14 in]
          }
          frame "Action: Change CSM Documentation Case to Front" {
            # "Your code here.\n(You can make a copy of, or modify, this frame)"
            n158 = String To Path(string=w405) -> (path=w406:path)
            n159 = Open VI Reference(vi path=w406) -> (vi reference=w385:refnum<vi>, error out=w384:errorcluster)  [unwired: 5 in]
            n160 = property class="VI"(reference=w385, error in=w384) -> (reference out=w388:refnum<vi>, error out=w387:errorcluster, "Diagram"=w386:refnum<vi>)
            n161 = property class="TopLvlDiag"(reference=w386, error in=w387) -> (error out=w391:errorcluster, "AllObjs[]"=w390:refnum<vi>[])  [unwired: 1 out]
            n162 = for {
              tunnel: w390 -> [w421] mode=indexing
              tunnel: w391 -> [w419]
              tunnel: [w418] -> w400
              tunnel: [w417] -> w399
              stop <- w417 continue-if-true
              w420 = refnum<vi> refnum  # WhileLoop
              n163 = To More Specific Class(target class=w420, reference=w421, error in=w419) -> (specific class reference=w418:refnum<vi>, error out=w417:errorcluster)
            }
            n164 = property class="WLoop"(reference=w400, error in=w399) -> (error out=w401:errorcluster, "Diagram.AllObjs[]"=w403:refnum<vi>[])  [unwired: 1 out]
            n165 = for {
              tunnel: w403 -> [w416] mode=indexing
              tunnel: w401 -> [w414]
              tunnel: [w413] -> w395
              tunnel: [w412] -> w394
              stop <- w412 continue-if-true
              w415 = refnum<vi> refnum  # CaseStructure
              n166 = To More Specific Class(target class=w415, reference=w416, error in=w414) -> (specific class reference=w413:refnum<vi>, error out=w412:errorcluster)
            }
            n167 = property class="CaseSel" props=["FrameNames", "Selector"](reference=w395, error in=w394) -> (reference out=w397:refnum<vi>, error out=w396:errorcluster, "FrameNames"=w392:string[])  [unwired: 1 out]
            n168 = Search 1D Array(1D array=w392, element=" \"CSM Documentation\" " ("y")) -> (index of element=w398:i32)  [unwired: 1 in]
            n169 = property class="CaseSel"(reference=w397, error in=w396, "VisFrame"=w398) -> (error out=w402:errorcluster)  [unwired: 1 out]
            n170 = Close Reference(reference=w403, error in (no error)=w402) -> (error out=w404:errorcluster)
            n171 = Close Reference(reference=w390, error in (no error)=w404) -> (error out=w389:errorcluster)
            n172 = invoke class="VI" method="Save.Instrument"(reference=w388, error in=w389) -> (reference out=w382:refnum<vi>, error out=w383:errorcluster)  [unwired: 4 in, 4 out]
            n173 = Close Reference(reference=w382, error in (no error)=w383) -> (error out=w407:errorcluster)
            n174 = call <vilib>:"Clear Errors.vi"("error in (no error)"=w407) -> ()  [unwired: 5 in, 2 out]
            n175 = call <vilib>:"Add State(s) to Queue__JKI_lib_State_Machine.vi"("State(s) in (\"\")"=w411) -> ("States Out"=w410:string)  [unwired: 14 in]
          }
        }
      }
    }
  }
  "error out" <- errorcluster {"status"=FALSE, "code"=0, "source"=""} ("error out")
